vi "Vision AE.vi"(7 "Update":bool, 11 "Vision Cluster (in)":T1) -> (3 "Vision Cluster (out)":T1)   [LabVIEW 2023]
uses:
  Vision Cluster Type Def.ctl
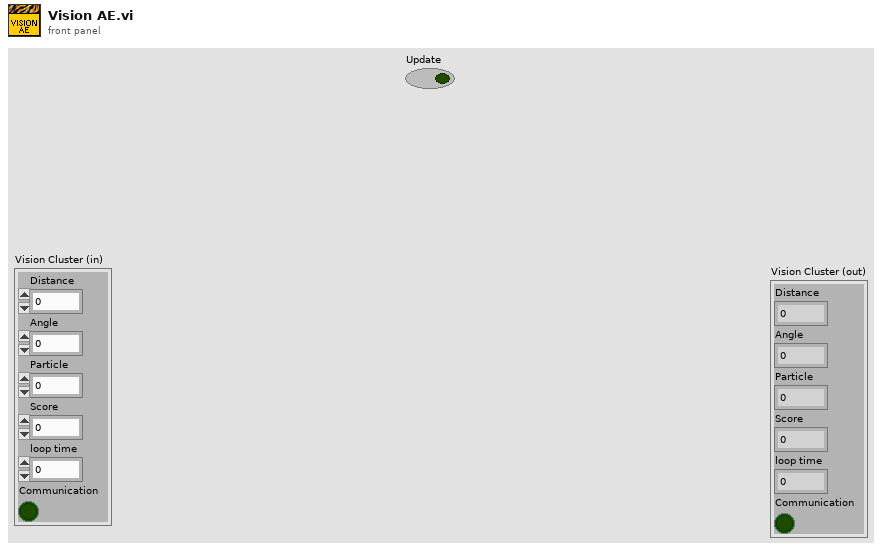
[diagram p1: front panel]
types:
  T1 = typedef "Vision Cluster Type Def.ctl" = cluster{"Distance":dbl, "Angle":dbl, "Particle":dbl, "Score":dbl, "loop time":dbl, "Communication":bool}
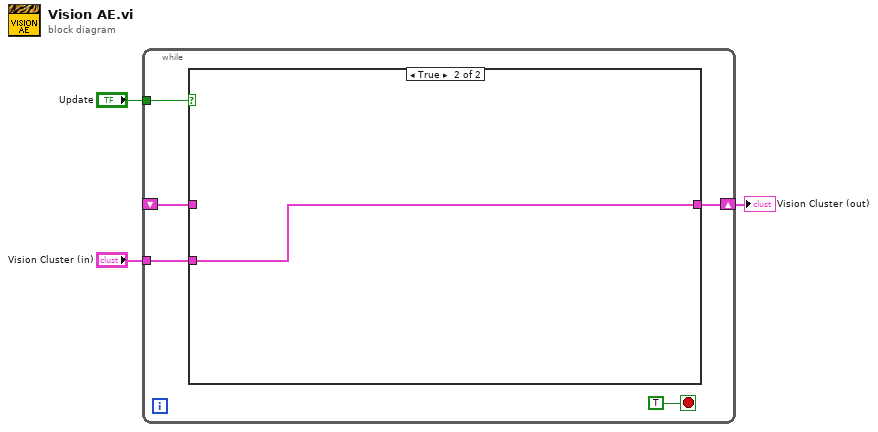
[diagram p0: block diagram]
diagram:
  n1 = while {
    shift-right: [w5] -> w1
    shift-left: _ -> [w6]
    tunnel: "Vision Cluster (in)" -> [w8]
    tunnel: "Update" -> [w7]
    stop <- TRUE stop-if-true
    n2 = case shown="True" w7 {
      tunnel: w8 -> [_ w10]
      tunnel: w6 -> [w9 _]
      tunnel: [w9 w10] -> w5
      frame False {
      }
      frame True {
      }
    }
  }
  "Vision Cluster (out)" <- w1
